vi "Correct Flow Rate and Get Dilution Factors.vi"(7 "Qbank":sgl, 8 "error in":errorcluster, 9 "RHbank":sgl, 10 "Qpurge":sgl, 11 "CRDS Cell in":refnum<class "CRDS Cell.lvclass">) -> (0 "error out":errorcluster, 3 "CRDS Cell out":refnum<class "CRDS Cell.lvclass">)   [LabVIEW 2014, in "CRDS Lib.lvlib" / "CRDS Cell.lvclass"]
doc: "Calculate the cell relative properties. RH and flow rates will be measured only one time for each cell bank and therefore we need to account for dilution. In addition, the extinction will be affected by the purge flows and must be accounted for in each cell. \n\nBoth the RH and flow rates are based on the relative volume of air associated with the bulk and purge flows and therefore have the same dilution factor. The assumption is that the RH in a particular cell will be affected only by the upstream purge flows. This assumption is correct given that diffusion is slow relative to the length of the cells."
uses:
  CRDS Cell.lvclass
  CRDS Cell.lvclass/CRDS Cell.ctl
  Data/Cell/Read hkParam.vi
  Data/Cell/Write hkParam.vi
  Data/Cell/CRDS Cell Data.lvclass
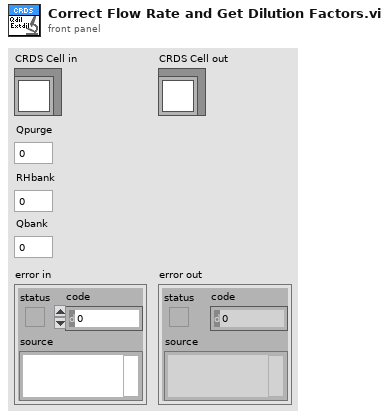
[diagram p1: front panel]
types:
  T1 = typedef "Base CRDS Lib.lvlib/calData.ctl" = cluster{"rhDilFac":sgl, "Q":sgl, "Tmean":sgl, "extDilFac":sgl, "rhCell":sgl, "P":sgl, "T":sgl}
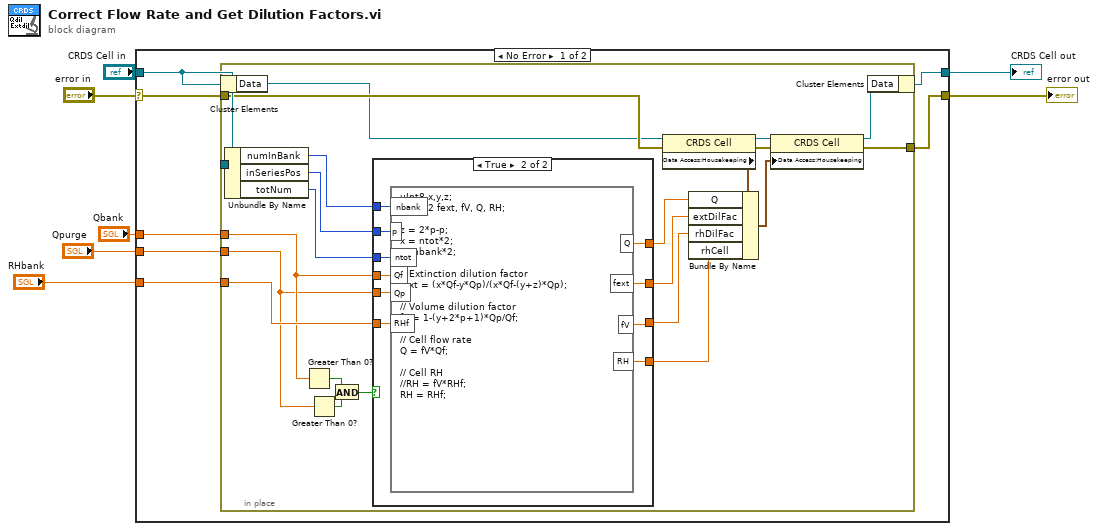
[diagram p0: block diagram]
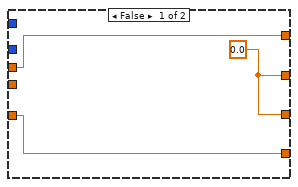
[diagram p2: hidden frame]
diagram:
  n1 = case shown="No Error" "error in" {
    selector: "error in" -> [w14 w51]
    tunnel: [w13 w51] -> w6
    tunnel: [w8 w50] -> w4
    tunnel: "CRDS Cell in" -> [w9 w50]
    tunnel: "Qpurge" -> [w10 _]
    tunnel: "Qbank" -> [w11 _]
    tunnel: "RHbank" -> [w12 _]
    frame No Error {
      n2 = in-place {
        in-place-border: w9 -> [w33]
        in-place-border: w14 -> [w32]
        in-place-border: [w30] -> w13
        in-place-border: w12 -> [w22]
        in-place-border: w11 -> [w21]
        in-place-border: w10 -> [w20]
        n3 = in-place-cluster #1(w9) -> ("Data"=w16:refnum<class "CRDS Cell Data.lvclass">)
        n4 = Unbundle By Name(w33) -> ("numInBank"=w28:u8, "inSeriesPos"=w27:u8, "totNum"=w29:u8)
        n5 = Greater Than 0?(x=w21) -> (x > 0?=w18:bool)
        n6 = Greater Than 0?(x=w20) -> (x > 0?=w19:bool)
        n7 = And(x=w18, y=w19) -> (x .and. y?=w17:bool)
        n8 = case shown="True" w17 {
          tunnel: w29 -> [_ w49]
          tunnel: w21 -> [w39 w48]
          tunnel: w28 -> [_ w47]
          tunnel: w27 -> [_ w46]
          tunnel: [w38 w45] -> w26
          tunnel: [w38 w44] -> w25
          tunnel: [w39 w43] -> w24
          tunnel: w20 -> [_ w42]
          tunnel: [w37 w41] -> w23
          tunnel: w22 -> [w37 w40]
          frame False {
            w38 = sgl 0.0
          }
          frame True {
            n9 = formula code="uInt8 x,y,z;\nfloat32 fext, fV, Q, RH;\n\nz = 2*p-p;\nx = ntot*2;\ny=nbank*2;\n\n// Extinction dilution factor\nfext = (x*Qf-y*Qp)/(x*Qf-(y+z)*Qp);\n\n// Volume dilution factor\nfV = 1-(y+2*p+1)*Qp/Qf;\n\n// Cell flow rate\nQ = fV*Qf;\n\n// Cell RH\n//RH = fV*RHf;\nRH = RHf;"("nbank"=w47, "p"=w46, "ntot"=w49, "Qf"=w48, "Qp"=w42, "RHf"=w40) -> ("fext"=w45:sgl, "fV"=w44:sgl, "Q"=w43:sgl, "RH"=w41:sgl)
          }
        }
        n10 = property class="CRDS Cell"(reference=w16, error in=w32) -> (reference out=w35:refnum<class "CRDS Cell Data.lvclass">, error out=w31:errorcluster, "Data Access:Housekeeping"=w36:T1)
        n11 = Bundle By Name(cluster=w36, "Q"=w24, "extDilFac"=w26, "rhDilFac"=w25, "rhCell"=w23) -> (w34:T1)
        n12 = property class="CRDS Cell"(reference=w35, error in=w31, "Data Access:Housekeeping"=w34) -> (reference out=w15:refnum<class "CRDS Cell Data.lvclass">, error out=w30:errorcluster)
        n13 = in-place-cluster #1("Data"=w15) -> (w8:refnum<class "CRDS Cell.lvclass">)
      }
    }
    frame Error {
    }
  }
  "error out" <- w6
  "CRDS Cell out" <- w4
